vi "Prepare to Wire Two Nodes.vi"(8 "error in (no error)":errorcluster, 10 "Nodes":refnum<vi>[](array[refnum]), 11 "Available Non-Nodes in":T1[](array[typedef])) -> (0 "error out":errorcluster, 2 "dup Nodes":refnum<vi>[](array[refnum]), 3 "Available Non-Nodes out":T1[](array[typedef]))   [LabVIEW 2016]
uses:
  <resource>/dialog/QuickDrop/plugins/_WireMultipleSupport/Available Non-Node.ctl
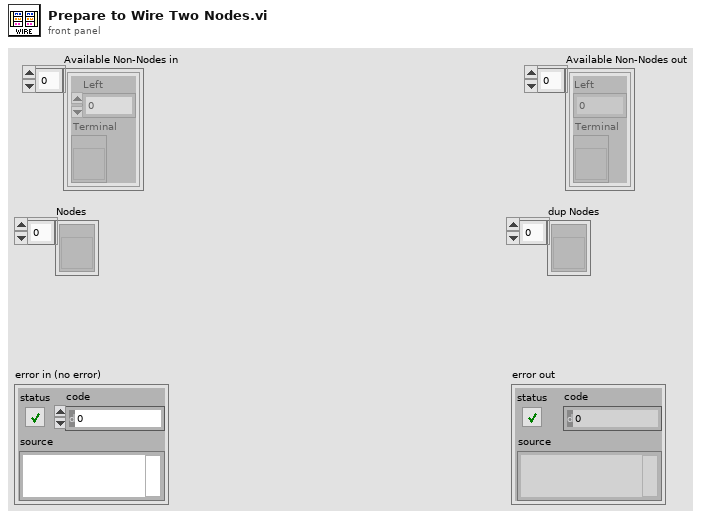
[diagram p1: front panel]
types:
  T1 = typedef "Available Non-Node.ctl" = cluster{"Left":i32, "Terminal":refnum<vi>}
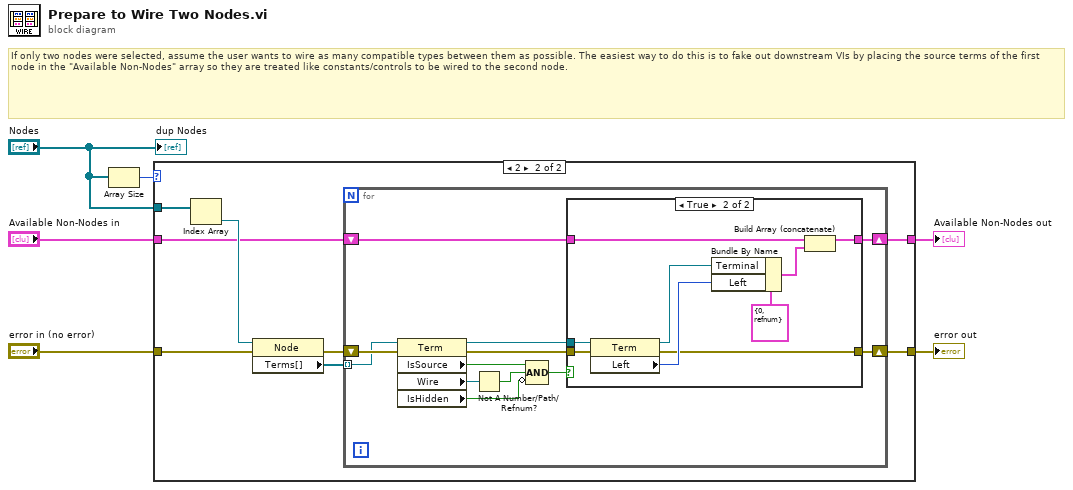
[diagram p0: block diagram]
diagram:
  # "If only two nodes were selected, assume the user wants to wire as many compatible types between them as possible. The easiest way to do this is to fake out downstream VIs by placing the source terms of the first node in the \"Available Non-Nodes\" array so they are treated like constants/controls to be wired to the second node."
  n1 = Array Size(array="Nodes") -> (size(s)=w6:i32)
  n2 = case shown="2" w6 {
    tunnel: "Available Non-Nodes in" -> [w8 w10]
    tunnel: "error in (no error)" -> [w7 w15]
    tunnel: "Nodes" -> [_ w16]
    tunnel: [w8 w9] -> w2
    tunnel: [w7 w12] -> w1
    frame Default {
    }
    frame 2 {
      n3 = Index Array(array=w16) -> (element=w14:refnum<vi>)  [unwired: 1 in]
      n4 = property class="Node"(reference=w14, error in=w15) -> (error out=w13:errorcluster, "Terms[]"=w11:refnum<vi>[])  [unwired: 1 out]
      n5 = for {
        shift-right: [w19] -> w12
        shift-left: w13 -> [w27]
        tunnel: w11 -> [w26] mode=indexing
        shift-right: [w21] -> w9
        shift-left: w10 -> [w23]
        n6 = property class="Term"(reference=w26, error in=w27) -> (reference out=w18:refnum<vi>, error out=w20:errorcluster, "IsSource"=w25:bool, "Wire"=w28:refnum<vi>, "IsHidden"=w17:bool)
        n7 = Not A Number/Path/Refnum?(number/path/refnum=w28) -> (NaN/Path/Refnum?=w24:bool)
        n8 = Compound Arithmetic op=AND(w25, w24, invert w17) -> (w22:bool)
        n9 = case shown="True" w22 {
          tunnel: w23 -> [w30 w39]
          tunnel: [w30 w38] -> w21
          tunnel: w20 -> [w29 w35]
          tunnel: [w29 w31] -> w19
          tunnel: w18 -> [_ w34]
          frame False {
          }
          frame True {
            n10 = property class="Term"(reference=w34, error in=w35) -> (reference out=w33:refnum<vi>, error out=w31:errorcluster, "Left"=w32:i32)
            n11 = Bundle By Name(cluster=T1 {"Left"=0, "Terminal"=refnum}, "Terminal"=w33, "Left"=w32) -> (w36:T1)
            n12 = Build Array (concatenate)(w39, w36) -> (w38:T1[])
          }
        }
      }
    }
  }
  "error out" <- w1
  "Available Non-Nodes out" <- w2
  "dup Nodes" <- "Nodes"
